vi "Parse CD XML.vi"(8 "error in (no error)":errorcluster, 10 "Custom Device XML Schema":path, 11 "Custom Device XML":path) -> (0 "error out":errorcluster, 3 "Custom Device Information":T1 {"Dependencies"."Type" items=["Absolute", "ToBase", "ToCommonDocDir", "ToApplicationDataDir"]; "Driver VIs"."Type" items=["Absolute", "ToBase", "ToCommonDocDir", "ToApplicationDataDir"]; "Execution Mode" items=["Asynchronous", "InlineHWInterface", "InlineModelInterface", "InlineTimingandSync", "AsynchronousTimingandSync"]})   [LabVIEW 2020, in "VeriStand SLSC Scripting.lvlib"]
uses:
  VeriStand SLSC Scripting.lvlib
  Controls/Custom Device Information.ctl
  Controls/Dependent File Information.ctl
  <vilib>/NI VeriStand/Custom Device API/Custom Device Supported Target.ctl
  NationalInstruments.VeriStand.XMLReader
  <vilib>/NI VeriStand/Custom Device API/Custom Device API.lvlib
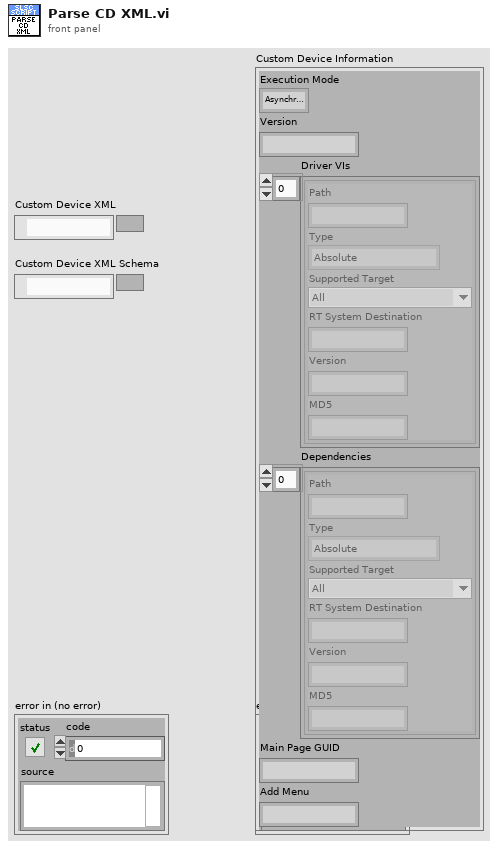
[diagram p1: front panel]
types:
  T1 = typedef "VeriStand SLSC Scripting.lvlib/Custom Device Information.ctl" = cluster{"Execution Mode":i32, "Version":string, "Driver VIs":T2[], "Dependencies":T2[], "Main Page GUID":string, "Add Menu":string}
  T2 = typedef "VeriStand SLSC Scripting.lvlib/Dependent File Information.ctl" = cluster{"Path":string, "Type":i32, "Supported Target":T3, "RT System Destination":string, "Version":string, "MD5":string}
  T3 = typedef "Custom Device API.lvlib/Custom Device Supported Target.ctl" = enum16{"All", "PharLap", "VxWorks", "Windows", "Linux_32_ARM", "Linux_x64", "PharLap & Windows", "PharLap & VxWorks", "VxWorks & Windows"}
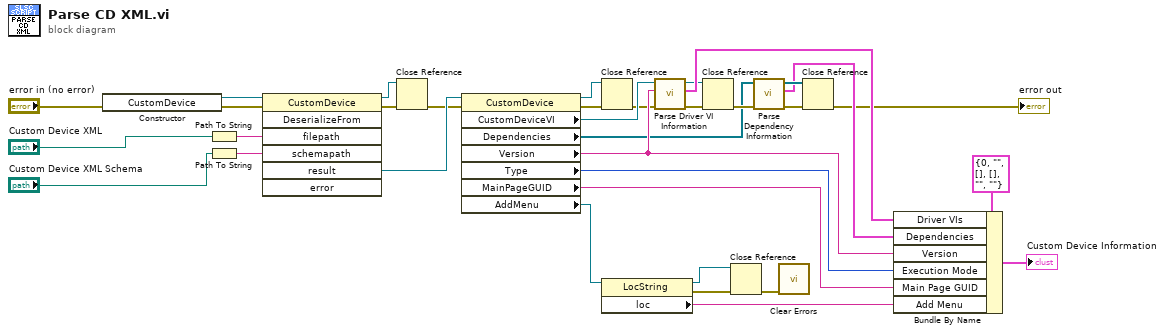
[diagram p0: block diagram]
diagram:
  n1 = constructor class="CustomDevice"(error in="error in (no error)") -> (reference out=w30:refnum<k24>, error out=w29:errorcluster)  [unwired: 2 in, 1 out]
  n2 = Path To String(path="Custom Device XML") -> (string=w33:string)
  n3 = Path To String(path="Custom Device XML Schema") -> (string=w31:string)
  n4 = invoke class="CustomDevice" method="DeserializeFrom"(reference=w30, error in=w29, "filepath"=w33, "schemapath"=w31) -> (reference out=w27:refnum<k24>, error out=w28:errorcluster, "result"=w26:refnum<k24>)  [unwired: 3 in, 4 out]
  n5 = Close Reference(reference=w27, error in (no error)=w28) -> (error out=w19:errorcluster)
  n6 = property class="CustomDevice"(reference=w26, error in=w19) -> (reference out=w17:refnum<k24>, error out=w25:errorcluster, "CustomDeviceVI"=w9:refnum<k24>, "Dependencies"=w5:refnum<k24>[], "Version"=w23:string, "Type"=w22:i32, "MainPageGUID"=w16:string, "AddMenu"=w15:refnum<k24>)
  n7 = Close Reference(reference=w17, error in (no error)=w25) -> (error out=w8:errorcluster)
  n8 = property class="LocString"(reference=w15) -> (reference out=w13:refnum<k24>, error out=w14:errorcluster, "loc"=w12:string)  [unwired: 1 in]
  n9 = call "Parse Driver VI Information.vi"("error in (no error)"=w8, "Version"=w23, "CustomDeviceVI"=w9) -> ("error out"=w18:errorcluster, "Driver VI Information"=w10:T2[], "CustomDeviceVI"=w7:refnum<k24>)  [unwired: 6 in]
  n10 = Close Reference(reference=w7, error in (no error)=w18) -> (error out=w6:errorcluster)
  n11 = Close Reference(reference=w13, error in (no error)=w14) -> (error out=w11:errorcluster)
  n12 = call "Parse Dependency Information.vi"("error in (no error)"=w6, "CustomDeviceVI"=w5) -> ("error out"=w4:errorcluster, "Dependency Information"=w2:T2[], "CustomDeviceVI"=w3:refnum<k24>[])  [unwired: 7 in]
  n13 = call <vilib>:"Clear Errors.vi"("error in (no error)"=w11) -> ()  [unwired: 5 in, 2 out]
  n14 = Close Reference(reference=w3, error in (no error)=w4) -> (error out=→"error out":errorcluster)
  n15 = Bundle By Name(cluster=T1 {"Execution Mode"=0, "Version"="", "Driver VIs"=[], "Dependencies"=[], "Main Page GUID"="", "Add Menu"=""} ("Custom Device Information"), "Driver VIs"=w10, "Dependencies"=w2, "Version"=w23, "Execution Mode"=w22, "Main Page GUID"=w16, "Add Menu"=w12) -> (→"Custom Device Information":T1)
